vi "Actor Core.vi"(8 "error in":errorcluster, 11 "TopUI in":refnum<class "TopUI.lvclass">) -> (0 "error out":errorcluster, 3 "Actor out":refnum<class "Actor.lvclass">)   [LabVIEW 2020, in "TopUI.lvlib" / "TopUI.lvclass"]
doc: "(<B>Filename</B>: Actor Framework.lvlib:Actor.lvclass:Actor Core.vi)\n\nReceives messages to the actor, reacts to them, and initiates any error handling that may shut the actor down.\n\nDescendant classes may override this VI to append parallel tasks for the actor to complete while it handles messages. Overrides use the Call Parent Class Method node."
uses:
  TopUI.lvclass
  <vilib>/ActorFramework/Actor/Actor.lvclass
  SimDaq/SimDaq/SimDaq.lvclass
  <vilib>/ActorFramework/Stop Msg/Stop Msg.lvclass
  TopUI Messages/CallDaqMeasure Msg/CallDaqMeasure Msg.lvclass
panel:
  in  "Measure":bool
  out "WGraph":waveform(dbl)(graph)
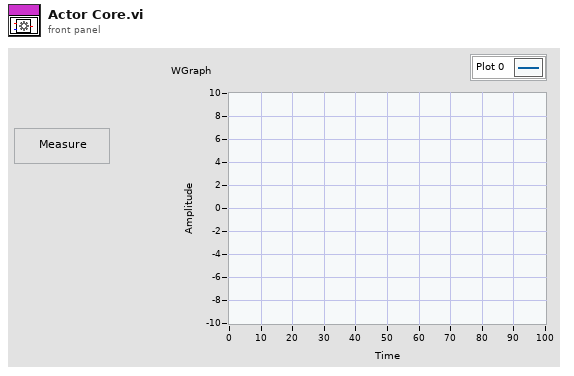
[diagram p1: front panel]
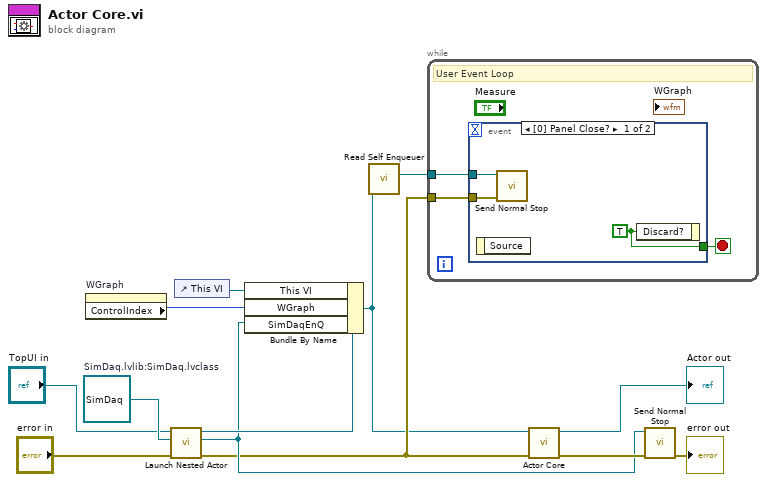
[diagram p0: block diagram]
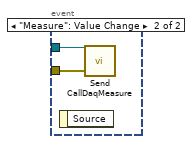
[diagram p2: hidden frame]
diagram:
  w9 = refnum<class "SimDaq.lvclass"> refnum  # SimDaq.lvlib:SimDaq.lvclass
  n1 = property on="WGraph" class="WFGraph (strict)"() -> ("ControlIndex"=w1:i32)  [unwired: 2 in, 2 out]
  n2 = call <vilib>:"Launch Nested Actor.vi"("error in (no error)"="error in", "Nested Actor"=w9, "Caller Actor in"="TopUI in") -> ("error out"=w5:errorcluster, "Nested Actor's Enqueuer"=w7:refnum<class "Message Enqueuer.lvclass">, "Caller Actor out"=w10:refnum<class "TopUI.lvclass">)  [unwired: 6 in]
  n3 = control-ref of="This VI"() -> (w2:refnum<vi>)
  n4 = Bundle By Name(cluster=w10, "This VI"=w2, "WGraph"=w1, "SimDaqEnQ"=w7) -> (w4:refnum<class "TopUI.lvclass">)
  n5 = call <vilib>:"Read Self Enqueuer.vi"("Actor"=w4) -> ("Self Enqueuer"=w3:refnum<class "Message Enqueuer.lvclass">)  [unwired: 10 in]
  n6 = while {
    tunnel: w5 -> [w15]
    tunnel: w3 -> [w14]
    stop <- w16 stop-if-true
    # "User Event Loop"
    n7 = event shown="[0] Panel Close?" {
      selector: _ -> [_ _]
      dyn-events: _ -> [_ _]
      timeout: _ -> [_ _]
      tunnel: [w19 _] -> w16
      tunnel: w15 -> [w18 w21]
      tunnel: w14 -> [w17 w20]
      event Panel Close? {
        w19 = TRUE ("Discard?")
        n8 = event-data() -> ()  [unwired: 1 in, 1 out]
        n9 = call <vilib>:"Send Normal Stop.vi"("error in (no error)"=w18, "Message Enqueuer"=w17) -> ()  [unwired: 9 in, 1 out]
        n10 = event-data("Discard?"=w19) -> ()  [unwired: 1 in, 1 out]
      }
      event "Measure": Value Change {
        n11 = event-data() -> ()  [unwired: 1 in, 1 out]
        n12 = call "Send CallDaqMeasure.vi"("error in (no error)"=w21, "Message Enqueuer"=w20) -> ()  [unwired: 8 in, 2 out]
      }
    }
  }
  n13 = call-parent "Actor Core.vi"("error in"=w5, "Actor in"=w4) -> ("error out"=w13:errorcluster, "Actor out"=→"Actor out":refnum<class "Actor.lvclass">)  [unwired: 8 in]
  n14 = call <vilib>:"Send Normal Stop.vi"("error in (no error)"=w13, "Message Enqueuer"=w7) -> ("error out"=→"error out":errorcluster)  [unwired: 9 in]
